vi "Read I-V Configuration.vi"(6 "RP I-V Configuration":T1={"I-V parameters"={"Start magnitude"=0.0, "Magnitude increment"=0.0, "End magnitude"=0.0, "Baseline length"=0, "Ramp length"=0, "Top  length"=0, "Threshold "=0.0, "Processing delay"=0, "Valhalla range"=0.0, "Interpolation"=0}, "Ranges"=[], "Pre-trigger duration"=0.01, "Post-trigger duration"=0.1, "Output delay"=0.1} {"Output delay" format="%#_6ps"; "Post-trigger duration" format="%#_6ps"; "Pre-trigger duration" format="%#_6ps"; "Ranges" format="%#_6pV"; "I-V parameters"."Valhalla range" format="%#_6pA"; "I-V parameters"."Processing delay" format="%dpts"; "I-V parameters"."Threshold" format="%#_6pV"; "I-V parameters"."Top  length" format="%dpts"; "I-V parameters"."Ramp length" format="%dpts"; "I-V parameters"."Baseline length" format="%dpts"; "I-V parameters"."End magnitude" format="%#_6pA"; "I-V parameters"."Magnitude increment" format="%#_6pA"; "I-V parameters"."Start magnitude" format="%#_6pA"}, 7 "Prefix":string, 8 "Error In":errorcluster, 9 "channel name":string, 10 "group name":string, 11 "tdms file":refnum<k34>) -> (0 "Error Out":errorcluster, 1 "channel name out":string, 2 "group name out":string, 3 "tdms file out":refnum<k34>, 4 "RP I-V Configuration out":T1={"I-V parameters"={"Start magnitude"=0.0, "Magnitude increment"=0.0, "End magnitude"=0.0, "Baseline length"=0, "Ramp length"=0, "Top  length"=0, "Threshold "=0.0, "Processing delay"=0, "Valhalla range"=0.0, "Interpolation"=0}, "Ranges"=[], "Pre-trigger duration"=0.01, "Post-trigger duration"=0.1, "Output delay"=0.1} {"Output delay" format="%#_6ps"; "Post-trigger duration" format="%#_6ps"; "Pre-trigger duration" format="%#_6ps"; "Ranges" format="%#_6pV"; "I-V parameters"."Valhalla range" format="%#_6pA"; "I-V parameters"."Processing delay" format="%dpts"; "I-V parameters"."Threshold" format="%#_6pV"; "I-V parameters"."Top  length" format="%dpts"; "I-V parameters"."Ramp length" format="%dpts"; "I-V parameters"."Baseline length" format="%dpts"; "I-V parameters"."End magnitude" format="%#_6pA"; "I-V parameters"."Magnitude increment" format="%#_6pA"; "I-V parameters"."Start magnitude" format="%#_6pA"}, 5 "found":bool)   [LabVIEW 2016]
uses:
  RP I-V Configuration.ctl
  Waform generation/I-V parameters.ctl
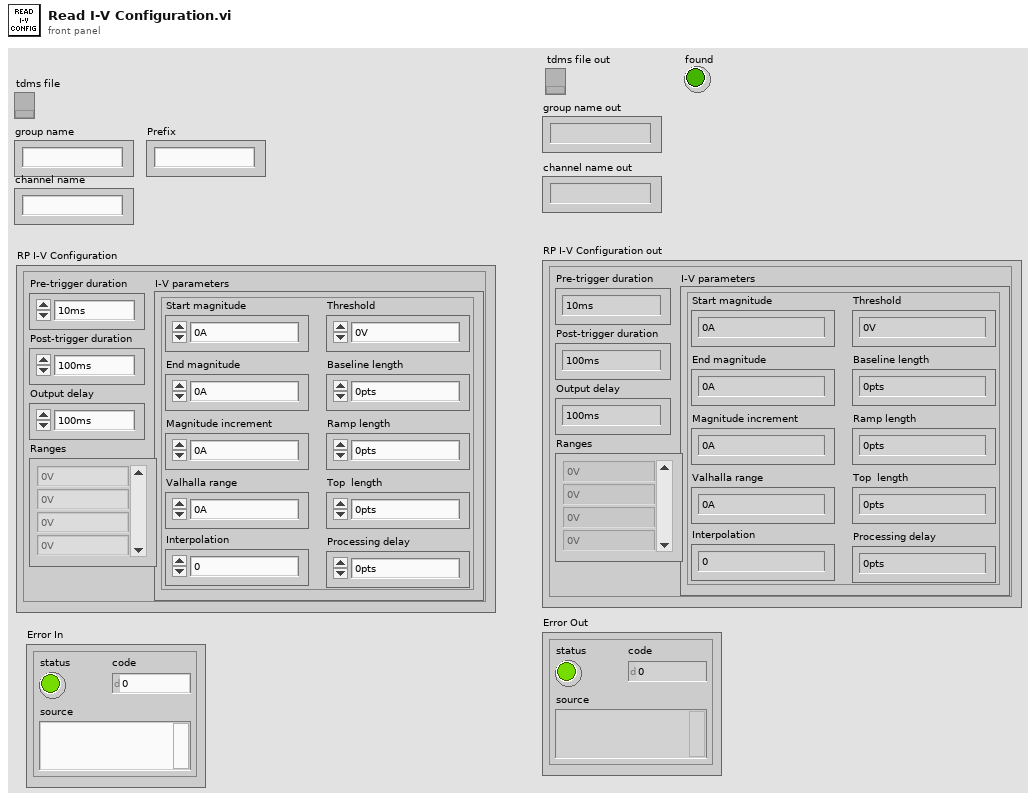
[diagram p1: front panel]
types:
  T1 = typedef "RP I-V Configuration.ctl" = cluster{"I-V parameters":T2, "Ranges":dbl[], "Pre-trigger duration":dbl, "Post-trigger duration":dbl, "Output delay":dbl}
  T2 = typedef "I-V parameters.ctl" = cluster{"Start magnitude":dbl, "Magnitude increment":dbl, "End magnitude":dbl, "Baseline length":i32, "Ramp length":i32, "Top  length":i32, "Threshold ":dbl, "Processing delay":u16, "Valhalla range":dbl, "Interpolation":i32}
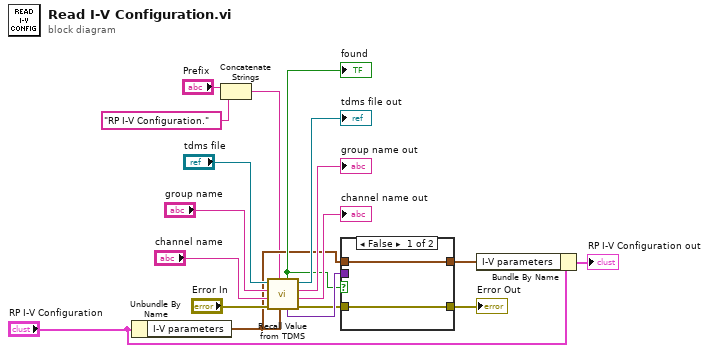
[diagram p0: block diagram]
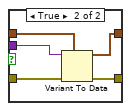
[diagram p2: hidden frame]
diagram:
  n1 = Unbundle By Name("RP I-V Configuration") -> ("I-V parameters"=w6:T2)
  n2 = Concatenate Strings("Prefix", "RP I-V Configuration." ("string")) -> (w2:string)
  n3 = call "Recall Value from TDMS.vi"("Value"=w6, "Prefix"=w2, "Error In"="Error In", "channel name"="channel name", "group name"="group name", "tdms file"="tdms file") -> ("Error Out"=w9:errorcluster, "channel name out"=→"channel name out":string, "group name out"=→"group name out":string, "tdms file out"=→"tdms file out":refnum<k34>, "Value out"=w11:variant, "found"=w10:bool)
  "found" <- w10
  n4 = case shown="False" w10 {
    tunnel: w11 -> [_ w25]
    tunnel: [w19 w24] -> w3
    tunnel: w9 -> [w20 w23]
    tunnel: [w20 w22] -> w8
    tunnel: w6 -> [w19 w21]
    frame False {
    }
    frame True {
      n5 = Variant To Data(error in=w23, type=w21, Variant=w25) -> (data=w24:T2, error out=w22:errorcluster)
    }
  }
  "Error Out" <- w8
  n6 = Bundle By Name(cluster="RP I-V Configuration", "I-V parameters"=w3) -> (→"RP I-V Configuration out":T1)
